vi "Format Button Message.vi"(7 "Switch":T1=enum."SW201 - My Cycle") -> (8 "Switch Message":string)   [LabVIEW 2018, in "2015 VA Washer.lvlib"]
uses:
  Projects/2015 VA Washer.lvlib
  type defs/UI Buttons.ctl
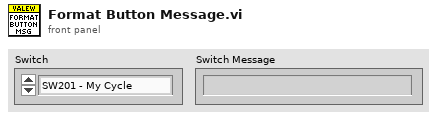
[diagram p1: front panel]
types:
  T1 = typedef "2015 VA Washer.lvlib/UI Buttons.ctl" = enum16{"Switch Off", "SW201 - My Cycle", "SW202 - Delay Wash", "SW203 - Extra Rinse", "SW204 - Signal / Volume", "SW205 - Spin", "SW206 - Deep Rinse / Fab Soft", "SW207 - Soil", "SW208 - Auto Soak", "SW209 - Temp", "SW210 - Warm Rinse", "SW211 - Deep Fill", "SW212 - Stain Remover", "SW213 - Power", "SW222 - Control Lock", "SW214 - Start / Pause", "SW301 - Start/Pause LE", "SW302 - Option Button LE"}
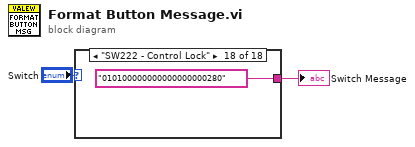
[diagram p0: block diagram]
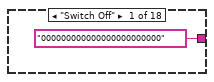
[diagram p2: hidden frame]
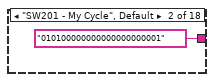
[diagram p3: hidden frame]
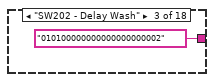
[diagram p4: hidden frame]
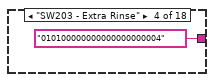
[diagram p5: hidden frame]
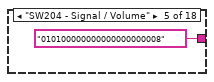
[diagram p6: hidden frame]
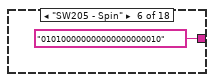
[diagram p7: hidden frame]
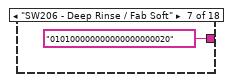
[diagram p8: hidden frame]
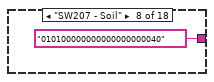
[diagram p9: hidden frame]
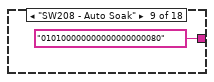
[diagram p10: hidden frame]
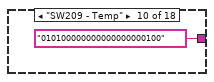
[diagram p11: hidden frame]
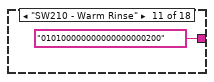
[diagram p12: hidden frame]
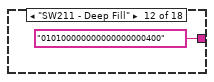
[diagram p13: hidden frame]
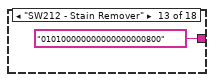
[diagram p14: hidden frame]
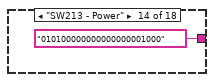
[diagram p15: hidden frame]
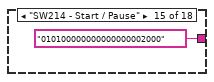
[diagram p16: hidden frame]
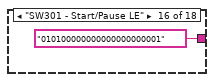
[diagram p17: hidden frame]
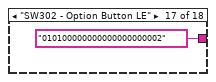
[diagram p18: hidden frame]
diagram:
  n1 = case shown="\"SW222 - Control Lock\"" "Switch" {
    tunnel: ["000000000000000000000000" ("Message") "010100000000000000000001" ("Message") "010100000000000000000002" ("Message") "010100000000000000000004" ("Message") "010100000000000000000008" ("Message") "010100000000000000000010" ("Message") "010100000000000000000020" ("Message") "010100000000000000000040" ("Message") "010100000000000000000080" ("Message") "010100000000000000000100" ("Message") "010100000000000000000200" ("Message") "010100000000000000000400" ("Message") "010100000000000000000800" ("Message") "010100000000000000001000" ("Message") "010100000000000000002000" ("Message") "010100000000000000000001" ("Message") "010100000000000000000002" ("Message") "010100000000000000000280" ("Message")] -> w1
    frame "Switch Off" {
    }
    frame "SW201 - My Cycle", Default {
    }
    frame "SW202 - Delay Wash" {
    }
    frame "SW203 - Extra Rinse" {
    }
    frame "SW204 - Signal / Volume" {
    }
    frame "SW205 - Spin" {
    }
    frame "SW206 - Deep Rinse / Fab Soft" {
    }
    frame "SW207 - Soil" {
    }
    frame "SW208 - Auto Soak" {
    }
    frame "SW209 - Temp" {
    }
    frame "SW210 - Warm Rinse" {
    }
    frame "SW211 - Deep Fill" {
    }
    frame "SW212 - Stain Remover" {
    }
    frame "SW213 - Power" {
    }
    frame "SW214 - Start / Pause" {
    }
    frame "SW301 - Start/Pause LE" {
    }
    frame "SW302 - Option Button LE" {
    }
    frame "SW222 - Control Lock" {
    }
  }
  "Switch Message" <- w1
